vi "ErrorLog Example.vi"() -> ()   [LabVIEW 2014]
uses:
  ErrorLog.lvclass
panel:
  out "Has Errors":bool
  in  "Clear Errors":bool
  in  "Show Dialog":bool
  in  "Ignore Duplicates?":bool
  in  "Log Error":bool
  in  "Error Context":string
  in  "Base Filename":string
  out "Log Files Stored At":path
  in  "Error to Log":errorcluster
  out "Log Files on Disk":string[][](table)
  # "This VI demonstrates the use of the Error Log library.\n\n    The MRU library is designed to quickly and easily automate synchronization of a 'Most Recently\nUsed' list between a System Combo Box and an INI file.\n\n    How to use this example:\n1. Set 'Base Filename' and 'Ignore Duplicates' as desired\n2. Run the VI\n3. Set the 'Error Context' and change the 'Error to Log'\n4. Click the 'Log Error' button\n5. Operate 'Dialog' and 'Clear' buttons\n6. Close the VI using the X (not the Stop/Abort button)"
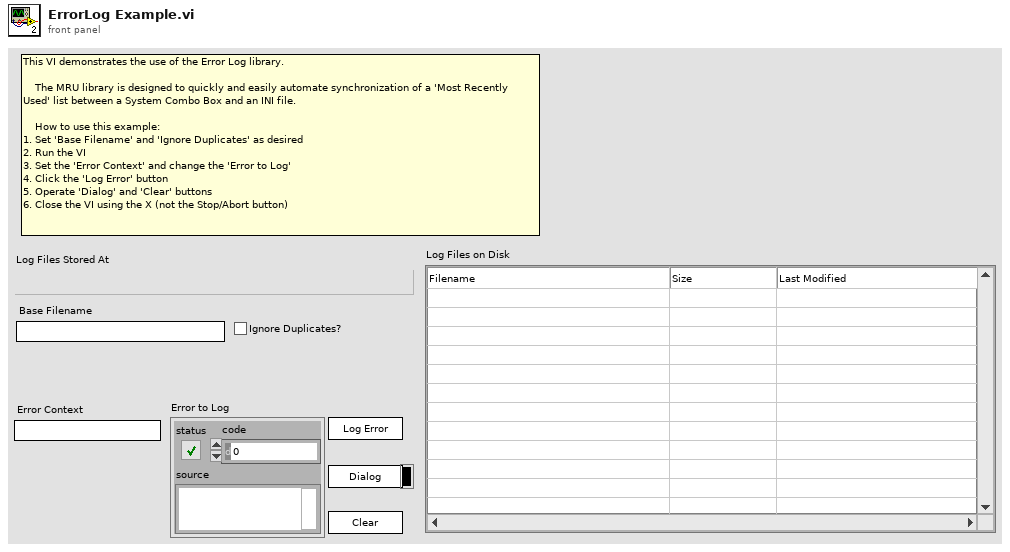
[diagram p1: front panel]
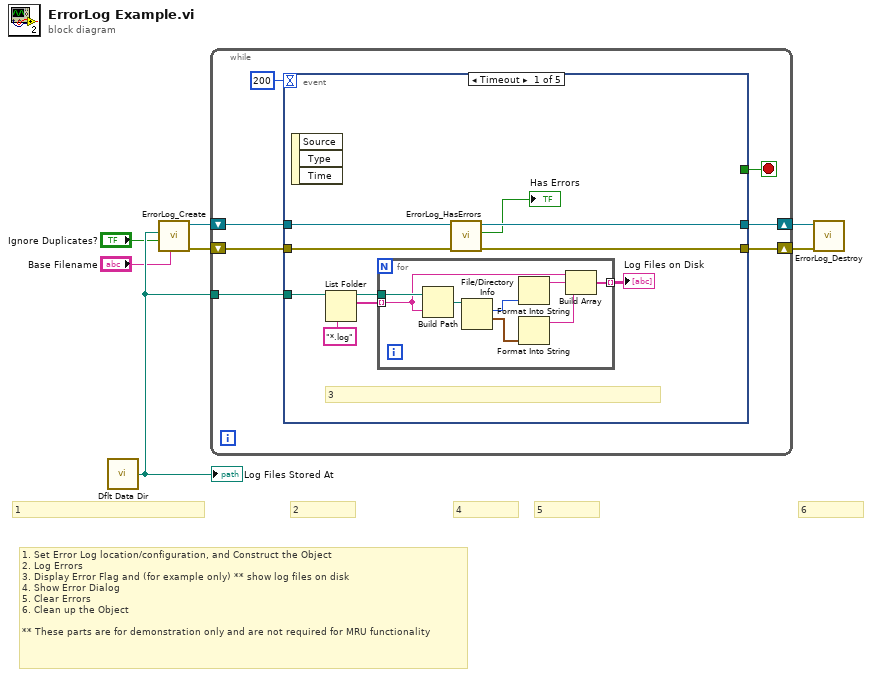
[diagram p0: block diagram]
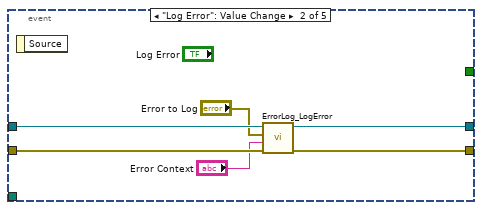
[diagram p2: hidden frame]
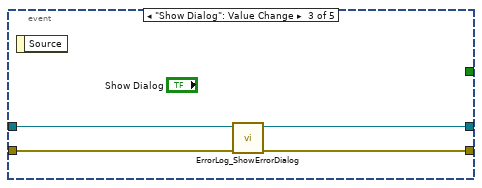
[diagram p3: hidden frame]
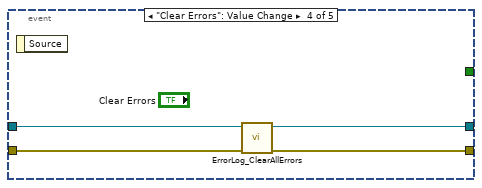
[diagram p4: hidden frame]
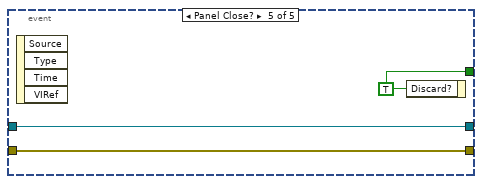
[diagram p5: hidden frame]
diagram:
  # "6"
  # "5"
  # "4"
  # "2"
  # "1"
  # "1. Set Error Log location/configuration, and Construct the Object\n2. Log Errors\n3. Display Error Flag and (for example only) ** show log files on disk\n4. Show Error Dialog\n5. Clear Errors\n6. Clean up the Object\n\n** These parts are for demonstration only and are not required for MRU functionality"
  n1 = call <vilib>:"Dflt Data Dir.vi"() -> ("App:Default Data Directory"=w3:path)
  "Log Files Stored At" <- w3
  n2 = call "ErrorLog_Create.vi"("ErrorLog FileName (\"Errors\")"="Base Filename", "Supress Consecutive Duplicates (T)"="Ignore Duplicates?", "ErrorLog Folder (c:\\)"=w3) -> ("error out"=w6:errorcluster, "reference out"=w7:refnum<class "ErrorLog.lvclass">)  [unwired: 7 in]
  n3 = while {
    tunnel: w3 -> [w12]
    shift-right: [w9] -> w5
    shift-left: w7 -> [w13]
    shift-right: [w8] -> w4
    shift-left: w6 -> [w11]
    stop <- w10 stop-if-true
    n4 = event shown="[0] Timeout" {
      selector: _ -> [_ _ _ _ _]
      dyn-events: _ -> [_ _ _ _ _]
      timeout: 200 -> [_ _ _ _ _]
      tunnel: w13 -> [w18 w38 w41 w45 w48]
      tunnel: w12 -> [w24 _ _ _ _]
      tunnel: w11 -> [w19 w36 w42 w46 w47]
      tunnel: [_ _ _ _ w49] -> w10
      tunnel: [w17 w37 w40 w44 w48] -> w9
      tunnel: [w16 w35 w39 w43 w47] -> w8
      event Timeout {
        # "3"
        n5 = event-data() -> ()  [unwired: 1 in, 3 out]
        n6 = List Folder(path=w24, pattern="*.log") -> (path out=w21:path, filenames=w22:string[])  [unwired: 2 in, 2 out]
        n7 = for {
          tunnel: w22 -> [w26] mode=indexing
          tunnel: w21 -> [w32]
          tunnel: [w25] -> w20 mode=indexing
          n8 = Build Path(base path=w32, name or relative path=w26) -> (appended path=w31:path)
          n9 = File/Directory Info(path=w31) -> (size=w30:i64, last mod=w29:timestamp)  [unwired: 1 in, 5 out]
          n10 = Format Into String(w30) -> (resulting string=w28:string)  [unwired: 3 in, 1 out]
          n11 = Format Into String(w29) -> (resulting string=w27:string)  [unwired: 3 in, 1 out]
          n12 = Build Array(w26, w28, w27) -> (w25:string[])
        }
        "Log Files on Disk" <- w20
        n13 = call-dynamic "ErrorLog_HasErrors.vi"("error in (no error)"=w19, "reference in"=w18) -> ("error out"=w16:errorcluster, "Has Errors"=→"Has Errors":bool, "reference out"=w17:refnum<class "ErrorLog.lvclass">)  [unwired: 7 in]
      }
      event "Log Error": Value Change {
        n14 = event-data() -> ()  [unwired: 1 in, 1 out]
        n15 = call-dynamic "ErrorLog_LogError.vi"("error in (no error)"=w36, "Context (\"Error\")"="Error Context", "Error To Log"="Error to Log", "reference in"=w38) -> ("error out"=w35:errorcluster, "reference out"=w37:refnum<class "ErrorLog.lvclass">)  [unwired: 3 in, 3 out]
      }
      event "Show Dialog": Value Change {
        n16 = event-data() -> ()  [unwired: 1 in, 1 out]
        n17 = call-dynamic "ErrorLog_ShowErrorDialog.vi"("error in (no error)"=w42, "reference in"=w41) -> ("error out"=w39:errorcluster, "reference out"=w40:refnum<class "ErrorLog.lvclass">)  [unwired: 8 in]
      }
      event "Clear Errors": Value Change {
        n18 = event-data() -> ()  [unwired: 1 in, 1 out]
        n19 = call-dynamic "ErrorLog_ClearAllErrors.vi"("error in (no error)"=w46, "reference in"=w45) -> ("error out"=w43:errorcluster, "reference out"=w44:refnum<class "ErrorLog.lvclass">)  [unwired: 8 in]
      }
      event Panel Close? {
        w49 = TRUE
        n20 = event-data() -> ()  [unwired: 1 in, 4 out]
        n21 = event-data("Discard?"=w49) -> ()  [unwired: 1 in, 1 out]
      }
    }
  }
  n22 = call-dynamic "ErrorLog_Destroy.vi"("error in (no error)"=w4, "reference in"=w5) -> ()  [unwired: 8 in, 2 out]
